vi "SumMatrix.vi"(8 "error in (no error)":errorcluster, 11 "matrix":T1) -> (0 "error out":errorcluster, 3 "Sum":dbl)   [LabVIEW 2017]
uses:
  <vilib>/Analysis/Matrix/Datatypes/RealMatrix.ctl
  <vilib>/Analysis/Matrix/NI_Matrix.lvlib
panel:
  out "matrix 2":T1
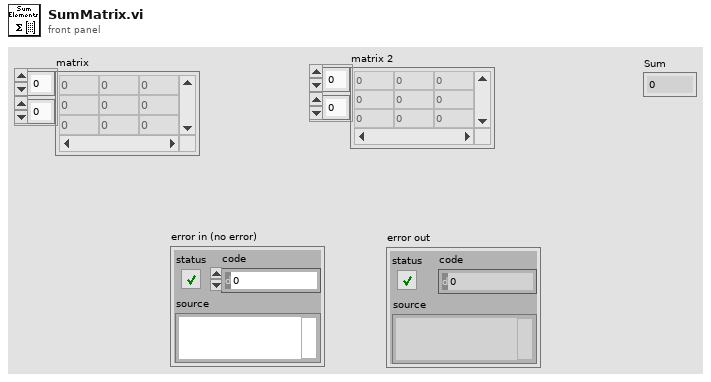
[diagram p1: front panel]
types:
  T1 = typedef "NI_Matrix.lvlib/RealMatrix.ctl" = dbl[][]
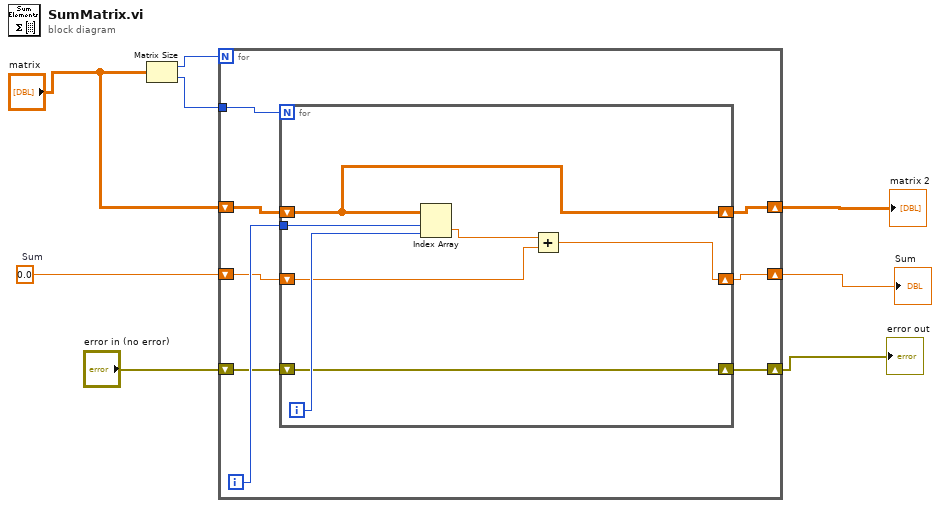
[diagram p0: block diagram]
diagram:
  w5 = 0.0  # Sum
  n1 = Matrix Size(0:"matrix") -> (1:w8:i32, 2:w7:i32)
  n2 = for {
    N: w8 -> [_]
    tunnel: w7 -> [w16]
    shift-right: [w13] -> w3
    shift-left: "matrix" -> [w14]
    shift-right: [w11] -> w4
    shift-left: w5 -> [w12]
    shift-right: [w10] -> w1
    shift-left: "error in (no error)" -> [w9]
    i -> [w15]
    n3 = for {
      N: w16 -> [_]
      tunnel: w15 -> [w22]
      shift-right: [w21] -> w13
      shift-left: w14 -> [w21]
      shift-right: [w18] -> w11
      shift-left: w12 -> [w19]
      shift-right: [w17] -> w10
      shift-left: w9 -> [w17]
      i -> [w23]
      n4 = Index Array(array=w21, index (row)=w22, index (col)=w23) -> (element=w20:dbl)
      n5 = Add(x=w20, y=w19) -> (x+y=w18:dbl)
    }
  }
  "Sum" <- w4
  "matrix 2" <- w3
  "error out" <- w1
